vi "TipsWhenDecodeCANdata.vi"(0 "ProgressBar":refnum<vi>, 1 "AllRowsNum":i32, 2 "i":i32, 5 "ProgressNum":refnum<vi>, 7 "Language":u32, 9 "Tips":refnum<vi>, 12 "MessageLinCnt":refnum<vi>, 13 "txtAllRowsNum":string, 14 "RowsLevel":i32) -> ()   [LabVIEW 2015]
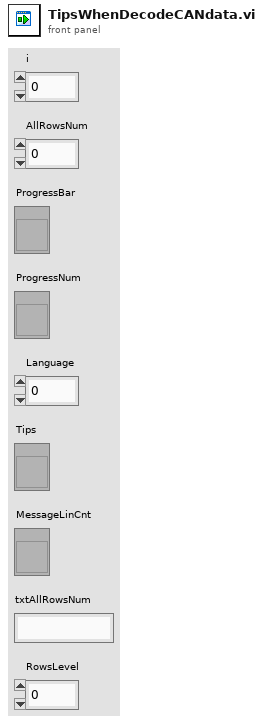
[diagram p1: front panel]
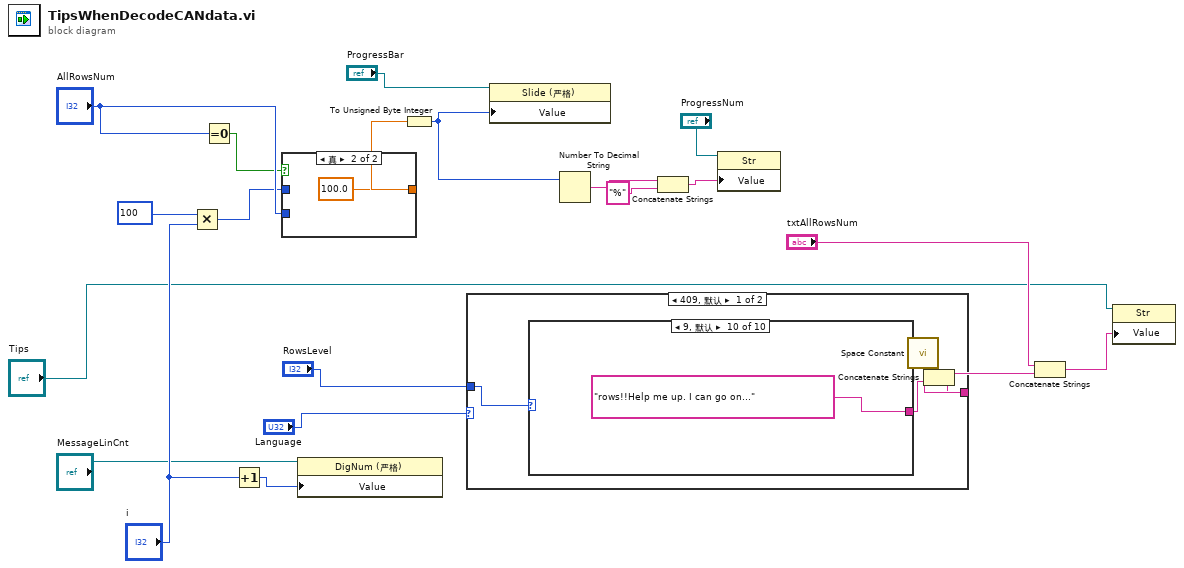
[diagram p0: block diagram]
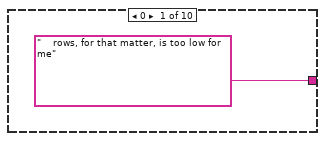
[diagram p2: hidden frame]
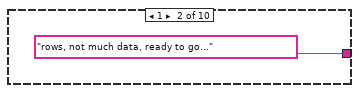
[diagram p3: hidden frame]
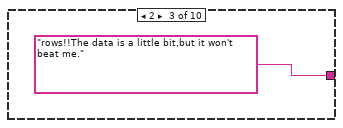
[diagram p4: hidden frame]
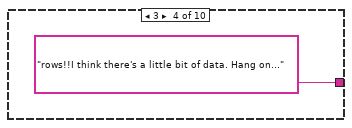
[diagram p5: hidden frame]
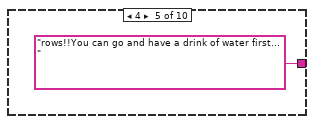
[diagram p6: hidden frame]
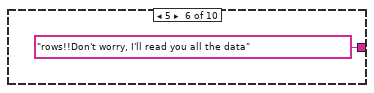
[diagram p7: hidden frame]
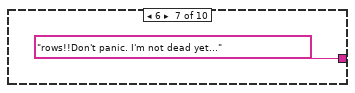
[diagram p8: hidden frame]
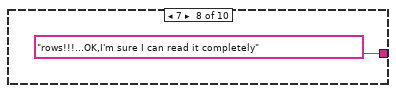
[diagram p9: hidden frame]
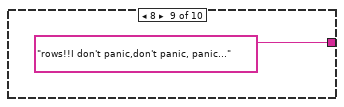
[diagram p10: hidden frame]
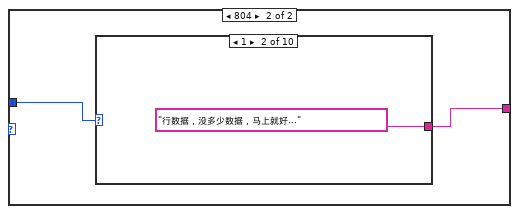
[diagram p11: hidden frame]
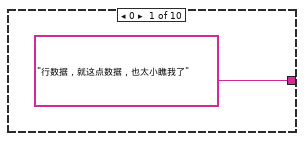
[diagram p12: hidden frame]
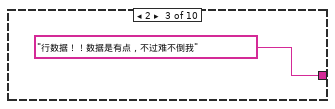
[diagram p13: hidden frame]
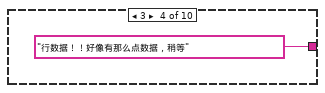
[diagram p14: hidden frame]
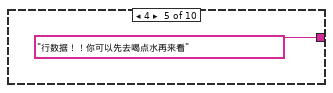
[diagram p15: hidden frame]
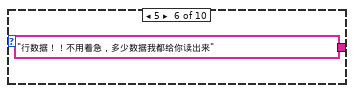
[diagram p16: hidden frame]
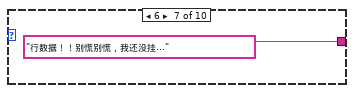
[diagram p17: hidden frame]
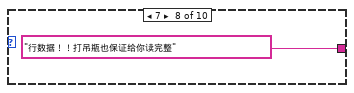
[diagram p18: hidden frame]
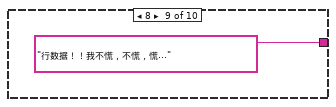
[diagram p19: hidden frame]
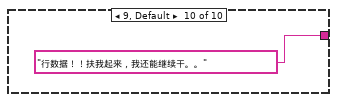
[diagram p20: hidden frame]
diagram:
  n1 = Multiply(x=100, y="i") -> (x*y=w2:i32)
  n2 = Equal To 0?(x="AllRowsNum") -> (x = 0?=w4:bool)
  n3 = Increment(x="i") -> (x+1=w16:i32)
  n4 = case shown="真" w4 {
    tunnel: w2 -> [w23 _]
    tunnel: "AllRowsNum" -> [w22 _]
    tunnel: [w21 100.0] -> w6
    frame False {
      n5 = Divide(x=w23, y=w22) -> (x/y=w21:dbl)
    }
    frame True {
    }
  }
  n6 = property class="DigNum (严格)"(reference="MessageLinCnt", "Value"=w16) -> ()  [unwired: 1 in, 2 out]
  n7 = To Unsigned Byte Integer(number=w6) -> (unsigned 8bit integer=w10:u8)
  n8 = case shown="409, 默认" "Language" {
    tunnel: "RowsLevel" -> [w28 w40]
    tunnel: [w26 w39] -> w19
    frame 409, Default {
      n9 = case shown="9, 默认" w28 {
        tunnel: ["    rows, for that matter, is too low for me" ("值") "rows, not much data, ready to go..." ("值") "rows!!The data is a little bit,but it won't beat me." ("值") "rows!!I think there's a little bit of data. Hang on..." ("值") "rows!!You can go and have a drink of water first..." ("值") "rows!!Don't worry, I'll read you all the data" ("值") "rows!!Don't panic. I'm not dead yet..." ("值") "rows!!!...OK,I'm sure I can read it completely" ("值") "rows!!I don't panic,don't panic, panic..." ("值") "rows!!Help me up. I can go on..." ("值")] -> w27
        frame 0 {
        }
        frame 1 {
        }
        frame 2 {
        }
        frame 3 {
        }
        frame 4 {
        }
        frame 5 {
        }
        frame 6 {
        }
        frame 7 {
        }
        frame 8 {
        }
        frame 9, Default {
        }
      }
      n10 = call <vilib>:"Space Constant.vi"() -> ("String"=w25:string)
      n11 = Concatenate Strings(w25, w27) -> (w26:string)
    }
    frame 804 {
      n12 = case shown="1" w40 {
        tunnel: ["行数据，就这点数据，也太小瞧我了" ("值") "行数据，没多少数据，马上就好..." ("值") "行数据！！数据是有点，不过难不倒我" ("值") "行数据！！好像有那么点数据，稍等" ("值") "行数据！！你可以先去喝点水再来看" ("值") "行数据！！不用着急，多少数据我都给你读出来" ("值") "行数据！！别慌别慌，我还没挂..." ("值") "行数据！！打吊瓶也保证给你读完整" ("值") "行数据！！我不慌，不慌，慌..." ("值") "行数据！！扶我起来，我还能继续干。。" ("值")] -> w39
        frame 0 {
        }
        frame 1 {
        }
        frame 2 {
        }
        frame 3 {
        }
        frame 4 {
        }
        frame 5 {
        }
        frame 6 {
        }
        frame 7 {
        }
        frame 8 {
        }
        frame 9, Default {
        }
      }
    }
  }
  n13 = property class="Slide (严格)"(reference="ProgressBar", "Value"=w10) -> ()  [unwired: 1 in, 2 out]
  n14 = Number To Decimal String(number=w10) -> (decimal integer string=w9:string)  [unwired: 1 in]
  n15 = Concatenate Strings(w9, "%" ("字符串")) -> (w8:string)
  n16 = property class="Str"(reference="ProgressNum", "Value"=w8) -> ()  [unwired: 1 in, 2 out]
  n17 = Concatenate Strings("txtAllRowsNum", w19) -> (w13:string)
  n18 = property class="Str"(reference="Tips", "Value"=w13) -> ()  [unwired: 1 in, 2 out]
